vi "Digio Write Protect.vi"(7 "Mask (0)":u32 max=16383, 8 "error in (no error)":errorcluster, 10 "Node In":string, 11 "VISA resource name":refnum<visa-resource-name>) -> (0 "error out":errorcluster, 2 "Node Out":string, 3 "VISA resource name out":refnum<visa-resource-name>, 4 "Command String":string)   [LabVIEW 2012, in "Keithley 2600 Series.lvlib"]
doc: "This VI creates a write protect mask that disables bits from being changed with the digio.writebit and digio.writeport functions.\n\nBits that are set to one cause the corresponding line to be write protected.\n\nThe binary equivalent of mask indicates the mask to be set for the I/O port. For exam­ple, a mask value of 7 has a binary equivalent 00000000000111. This mask write protects lines 1, 2 and 3.\n\n<b>Functions and Attributes Used</b>\ndigio.writeprotect\n\nNote:\nDigital IO feature is not supported with Keithley 2604B, 2614B, 2634B."
uses:
  Keithley 2600 Series.lvlib
  Private/GlobalVariables.vi
panel:
  # "(c) 2008 Keithley Instruments, Inc.  ALL RIGHTS RESERVED."
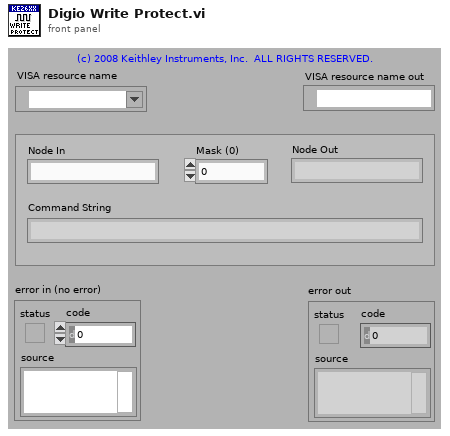
[diagram p1: front panel]
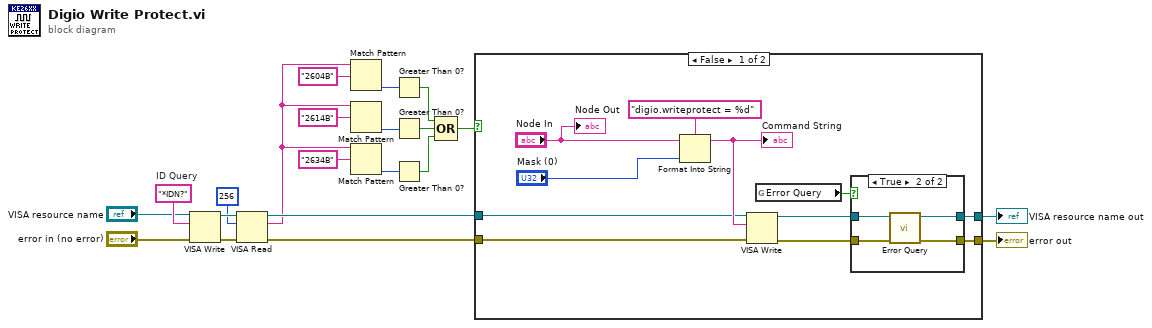
[diagram p0: block diagram]
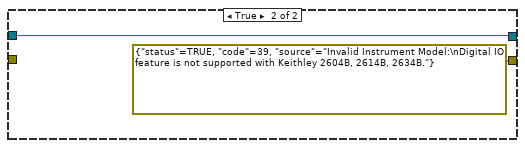
[diagram p3: hidden frame]
diagram:
  w16 = "*IDN?"  # ID Query
  n1 = VISA Write(VISA resource name="VISA resource name", write buffer=w16, error in (no error)="error in (no error)") -> (VISA resource name out=w19:refnum<visa-resource-name>, error out=w18:errorcluster)  [unwired: 1 out]
  n2 = VISA Read(VISA resource name=w19, byte count=u32 256, error in (no error)=w18) -> (VISA resource name out=w15:refnum<visa-resource-name>, read buffer=w1:string, error out=w14:errorcluster)  [unwired: 1 out]
  n3 = Match Pattern(string=w1, regular expression="2604B" ("y")) -> (offset past match=w8:i32)  [unwired: 1 in, 3 out]
  n4 = Match Pattern(string=w1, regular expression="2614B" ("y")) -> (offset past match=w7:i32)  [unwired: 1 in, 3 out]
  n5 = Match Pattern(string=w1, regular expression="2634B" ("y")) -> (offset past match=w6:i32)  [unwired: 1 in, 3 out]
  n6 = Greater Than 0?(x=w8) -> (x > 0?=w5:bool)
  n7 = Greater Than 0?(x=w7) -> (x > 0?=w4:bool)
  n8 = Greater Than 0?(x=w6) -> (x > 0?=w3:bool)
  n9 = Compound Arithmetic op=OR(w5, w4, w3) -> (w2:bool)
  n10 = case shown="False" w2 {
    tunnel: [w29 w40] -> w21
    tunnel: [w28 errorcluster {"status"=TRUE, "code"=39, "source"="Invalid Instrument Model:\nDigital IO feature is not supported with Keithley 2604B, 2614B, 2634B."} ("error out")] -> w20
    tunnel: w15 -> [w23 w40]
    tunnel: w14 -> [w22 _]
    frame False {
      n11 = Format Into String(format string="digio.writeprotect = %d", initial string="Node In", "Mask (0)") -> (resulting string=w24:string)  [unwired: 1 in, 1 out]
      "Command String" <- w24
      n12 = VISA Write(VISA resource name=w23, write buffer=w24, error in (no error)=w22) -> (VISA resource name out=w31:refnum<visa-resource-name>, error out=w30:errorcluster)  [unwired: 1 out]
      n13 = global read "GlobalVariables.vi" "Error Query"() -> (w32:bool)
      n14 = case shown="True" w32 {
        tunnel: w31 -> [w34 w38]
        tunnel: w30 -> [w33 w37]
        tunnel: [w34 w36] -> w29
        tunnel: [w33 w35] -> w28
        frame False {
        }
        frame True {
          n15 = call "Error Query.vi"("error in (no error)"=w37, "VISA resource name"=w38) -> ("error out"=w35:errorcluster, "VISA resource name out"=w36:refnum<visa-resource-name>)  [unwired: 8 out]
        }
      }
      "Node Out" <- "Node In"
    }
    frame True {
    }
  }
  "VISA resource name out" <- w21
  "error out" <- w20
